vi "test - all.vi"() -> ()   [LabVIEW 2020]
uses:
  ui-testing.lvlib
panel:
  in  "Start test14 (SSP)":bool
  in  "Start test14 (SP)":bool
  in  "Start test14":bool
  in  "Start test13":bool
  in  "Start test12":bool
  in  "Start test11":bool
  in  "Start test10":bool
  in  "Start test9":bool
  in  "Start test8":bool
  in  "Start test7":bool
  in  "Start test6":bool
  in  "Start test5":bool
  in  "Start test4b":bool
  in  "Start test4":bool
  in  "Start test3":bool
  in  "Start test2":bool
  in  "Start test1":bool
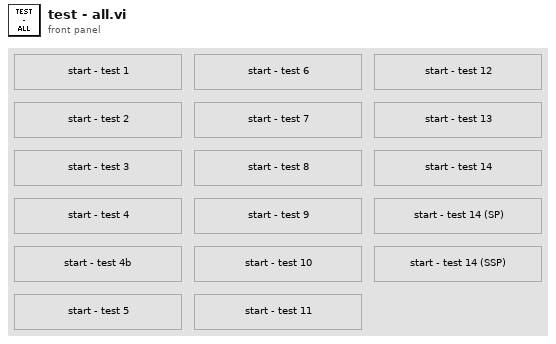
[diagram p1: front panel]
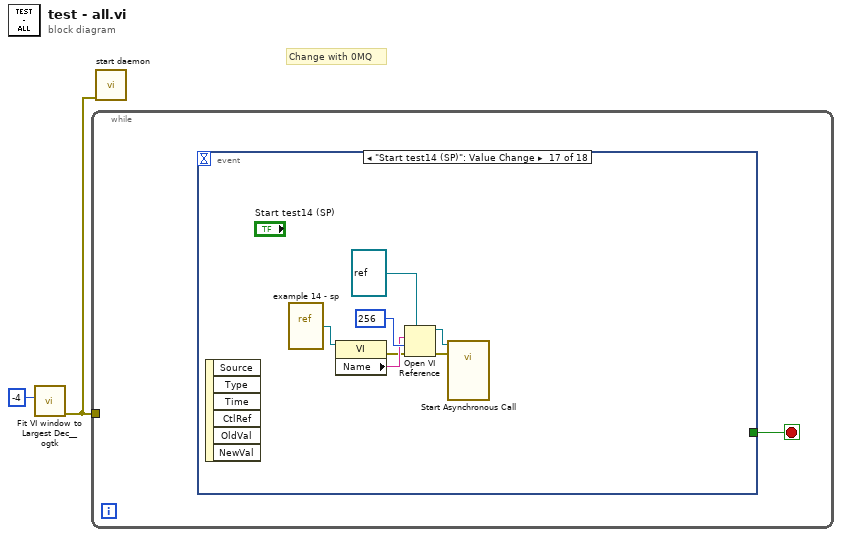
[diagram p0: block diagram]
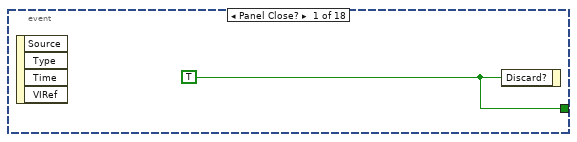
[diagram p2: hidden frame]
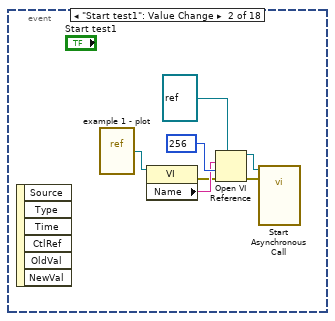
[diagram p3: hidden frame]
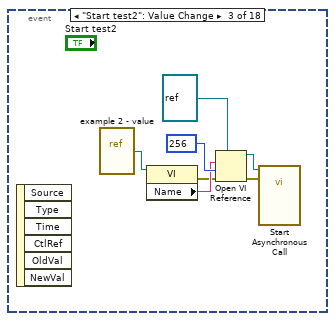
[diagram p4: hidden frame]
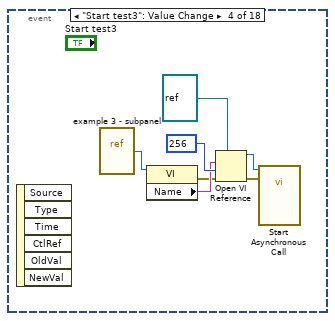
[diagram p5: hidden frame]
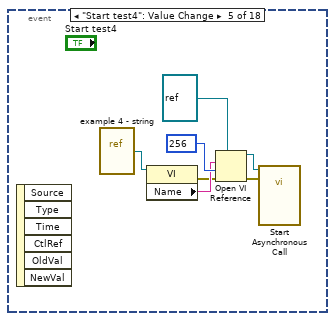
[diagram p6: hidden frame]
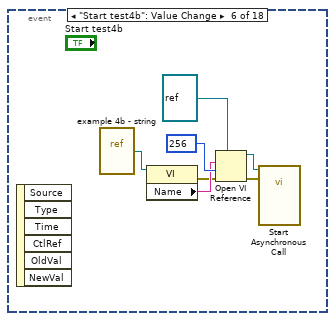
[diagram p7: hidden frame]
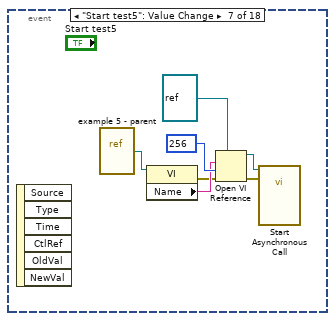
[diagram p8: hidden frame]
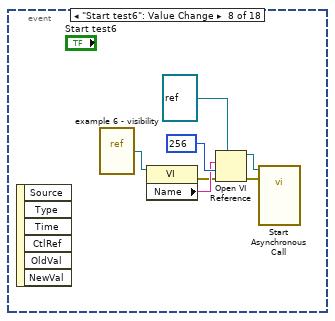
[diagram p9: hidden frame]
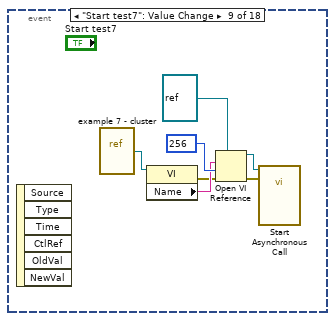
[diagram p10: hidden frame]
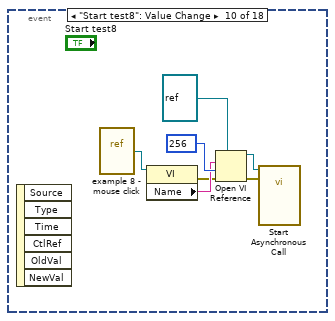
[diagram p11: hidden frame]
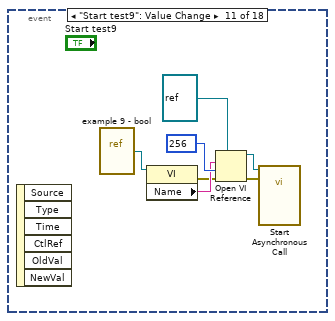
[diagram p12: hidden frame]
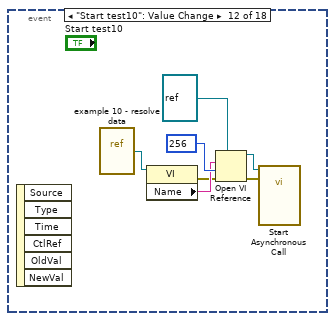
[diagram p13: hidden frame]
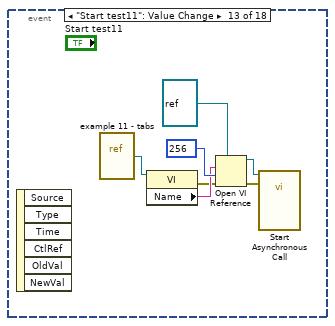
[diagram p14: hidden frame]
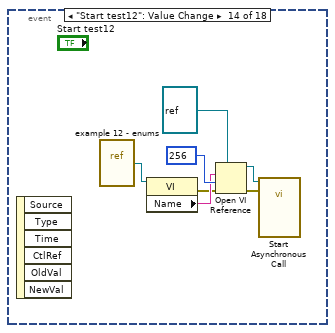
[diagram p15: hidden frame]
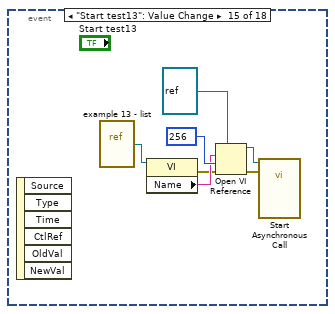
[diagram p16: hidden frame]
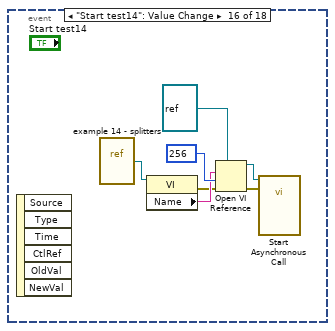
[diagram p17: hidden frame]
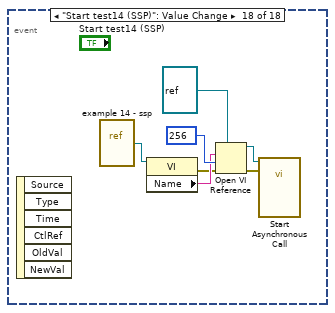
[diagram p18: hidden frame]
diagram:
  # "Change with 0MQ"
  n1 = call <userlib>:"Fit VI window to Largest Dec__ogtk.vi"("border spacing (2 px)"=-4) -> ("error out"=w1:errorcluster)  [unwired: 5 in, 1 out]
  n2 = while {
    tunnel: w1 -> [_]
    stop <- w3 stop-if-true
    n3 = event shown="[16] \"Start test14 (SP)\": Value Change" {
      selector: _ -> [_ _ _ _ _ _ _ _ _ _ _ _ _ _ _ _ _ _]
      dyn-events: _ -> [_ _ _ _ _ _ _ _ _ _ _ _ _ _ _ _ _ _]
      timeout: _ -> [_ _ _ _ _ _ _ _ _ _ _ _ _ _ _ _ _ _]
      tunnel: [w4 _ _ _ _ _ _ _ _ _ _ _ _ _ _ _ _ _] -> w3
      event Panel Close? {
        w4 = TRUE
        n4 = event-data() -> ()  [unwired: 1 in, 4 out]
        n5 = event-data("Discard?"=w4) -> ()  [unwired: 1 in, 1 out]
      }
      event "Start test1": Value Change {
        n6 = event-data() -> ()  [unwired: 1 in, 6 out]
        n7 = vi-ref "example 1 - plot.vi"() -> (w7:refnum<vi>)
        n8 = property class="VI"(reference=w7) -> (error out=w5:errorcluster, "Name"=w6:string)  [unwired: 1 in, 1 out]
        n9 = Open VI Reference(type specifier VI Refnum (for type only)=refnum<vi> refnum, vi path=w6, options=256 ("call and forget"), error in (no error)=w5) -> (vi reference=w9:refnum<vi>, error out=w8:errorcluster)  [unwired: 2 in]
        n10 = call-by-ref "Start Asynchronous Call"(reference=w9, error in=w8) -> ()  [unwired: 12 in, 2 out]
      }
      event "Start test2": Value Change {
        n11 = event-data() -> ()  [unwired: 1 in, 6 out]
        n12 = vi-ref "example 2 - value.vi"() -> (w14:refnum<vi>)
        n13 = property class="VI"(reference=w14) -> (error out=w12:errorcluster, "Name"=w13:string)  [unwired: 1 in, 1 out]
        n14 = Open VI Reference(type specifier VI Refnum (for type only)=refnum<vi> refnum, vi path=w13, options=256 ("call and forget"), error in (no error)=w12) -> (vi reference=w16:refnum<vi>, error out=w15:errorcluster)  [unwired: 2 in]
        n15 = call-by-ref "Start Asynchronous Call"(reference=w16, error in=w15) -> ()  [unwired: 12 in, 2 out]
      }
      event "Start test3": Value Change {
        n16 = event-data() -> ()  [unwired: 1 in, 6 out]
        n17 = vi-ref "example 3 - subpanel.vi"() -> (w21:refnum<vi>)
        n18 = property class="VI"(reference=w21) -> (error out=w19:errorcluster, "Name"=w20:string)  [unwired: 1 in, 1 out]
        n19 = Open VI Reference(type specifier VI Refnum (for type only)=refnum<vi> refnum, vi path=w20, options=256 ("call and forget"), error in (no error)=w19) -> (vi reference=w23:refnum<vi>, error out=w22:errorcluster)  [unwired: 2 in]
        n20 = call-by-ref "Start Asynchronous Call"(reference=w23, error in=w22) -> ()  [unwired: 12 in, 2 out]
      }
      event "Start test4": Value Change {
        n21 = event-data() -> ()  [unwired: 1 in, 6 out]
        n22 = vi-ref "example 4 - string.vi"() -> (w28:refnum<vi>)
        n23 = property class="VI"(reference=w28) -> (error out=w26:errorcluster, "Name"=w27:string)  [unwired: 1 in, 1 out]
        n24 = Open VI Reference(type specifier VI Refnum (for type only)=refnum<vi> refnum, vi path=w27, options=256 ("call and forget"), error in (no error)=w26) -> (vi reference=w30:refnum<vi>, error out=w29:errorcluster)  [unwired: 2 in]
        n25 = call-by-ref "Start Asynchronous Call"(reference=w30, error in=w29) -> ()  [unwired: 12 in, 2 out]
      }
      event "Start test4b": Value Change {
        n26 = event-data() -> ()  [unwired: 1 in, 6 out]
        n27 = vi-ref "example 4b - string.vi"() -> (w35:refnum<vi>)
        n28 = property class="VI"(reference=w35) -> (error out=w33:errorcluster, "Name"=w34:string)  [unwired: 1 in, 1 out]
        n29 = Open VI Reference(type specifier VI Refnum (for type only)=refnum<vi> refnum, vi path=w34, options=256 ("call and forget"), error in (no error)=w33) -> (vi reference=w37:refnum<vi>, error out=w36:errorcluster)  [unwired: 2 in]
        n30 = call-by-ref "Start Asynchronous Call"(reference=w37, error in=w36) -> ()  [unwired: 12 in, 2 out]
      }
      event "Start test5": Value Change {
        n31 = event-data() -> ()  [unwired: 1 in, 6 out]
        n32 = vi-ref "example 5 - parent.vi"() -> (w42:refnum<vi>)
        n33 = property class="VI"(reference=w42) -> (error out=w40:errorcluster, "Name"=w41:string)  [unwired: 1 in, 1 out]
        n34 = Open VI Reference(type specifier VI Refnum (for type only)=refnum<vi> refnum, vi path=w41, options=256 ("call and forget"), error in (no error)=w40) -> (vi reference=w44:refnum<vi>, error out=w43:errorcluster)  [unwired: 2 in]
        n35 = call-by-ref "Start Asynchronous Call"(reference=w44, error in=w43) -> ()  [unwired: 12 in, 2 out]
      }
      event "Start test6": Value Change {
        n36 = event-data() -> ()  [unwired: 1 in, 6 out]
        n37 = vi-ref "example 6 - visibility.vi"() -> (w49:refnum<vi>)
        n38 = property class="VI"(reference=w49) -> (error out=w47:errorcluster, "Name"=w48:string)  [unwired: 1 in, 1 out]
        n39 = Open VI Reference(type specifier VI Refnum (for type only)=refnum<vi> refnum, vi path=w48, options=256 ("call and forget"), error in (no error)=w47) -> (vi reference=w51:refnum<vi>, error out=w50:errorcluster)  [unwired: 2 in]
        n40 = call-by-ref "Start Asynchronous Call"(reference=w51, error in=w50) -> ()  [unwired: 12 in, 2 out]
      }
      event "Start test7": Value Change {
        n41 = event-data() -> ()  [unwired: 1 in, 6 out]
        n42 = vi-ref "example 7 - cluster.vi"() -> (w56:refnum<vi>)
        n43 = property class="VI"(reference=w56) -> (error out=w54:errorcluster, "Name"=w55:string)  [unwired: 1 in, 1 out]
        n44 = Open VI Reference(type specifier VI Refnum (for type only)=refnum<vi> refnum, vi path=w55, options=256 ("call and forget"), error in (no error)=w54) -> (vi reference=w58:refnum<vi>, error out=w57:errorcluster)  [unwired: 2 in]
        n45 = call-by-ref "Start Asynchronous Call"(reference=w58, error in=w57) -> ()  [unwired: 12 in, 2 out]
      }
      event "Start test8": Value Change {
        n46 = event-data() -> ()  [unwired: 1 in, 6 out]
        n47 = vi-ref "example 8 - mouse click.vi"() -> (w63:refnum<vi>)
        n48 = property class="VI"(reference=w63) -> (error out=w61:errorcluster, "Name"=w62:string)  [unwired: 1 in, 1 out]
        n49 = Open VI Reference(type specifier VI Refnum (for type only)=refnum<vi> refnum, vi path=w62, options=256 ("call and forget"), error in (no error)=w61) -> (vi reference=w65:refnum<vi>, error out=w64:errorcluster)  [unwired: 2 in]
        n50 = call-by-ref "Start Asynchronous Call"(reference=w65, error in=w64) -> ()  [unwired: 12 in, 2 out]
      }
      event "Start test9": Value Change {
        n51 = event-data() -> ()  [unwired: 1 in, 6 out]
        n52 = vi-ref "example 9 - bool.vi"() -> (w70:refnum<vi>)
        n53 = property class="VI"(reference=w70) -> (error out=w68:errorcluster, "Name"=w69:string)  [unwired: 1 in, 1 out]
        n54 = Open VI Reference(type specifier VI Refnum (for type only)=refnum<vi> refnum, vi path=w69, options=256 ("call and forget"), error in (no error)=w68) -> (vi reference=w72:refnum<vi>, error out=w71:errorcluster)  [unwired: 2 in]
        n55 = call-by-ref "Start Asynchronous Call"(reference=w72, error in=w71) -> ()  [unwired: 12 in, 2 out]
      }
      event "Start test10": Value Change {
        n56 = event-data() -> ()  [unwired: 1 in, 6 out]
        n57 = vi-ref "example 10 - resolve data.vi"() -> (w77:refnum<vi>)
        n58 = property class="VI"(reference=w77) -> (error out=w75:errorcluster, "Name"=w76:string)  [unwired: 1 in, 1 out]
        n59 = Open VI Reference(type specifier VI Refnum (for type only)=refnum<vi> refnum, vi path=w76, options=256 ("call and forget"), error in (no error)=w75) -> (vi reference=w79:refnum<vi>, error out=w78:errorcluster)  [unwired: 2 in]
        n60 = call-by-ref "Start Asynchronous Call"(reference=w79, error in=w78) -> ()  [unwired: 12 in, 2 out]
      }
      event "Start test11": Value Change {
        n61 = event-data() -> ()  [unwired: 1 in, 6 out]
        n62 = vi-ref "example 11 - tabs.vi"() -> (w84:refnum<vi>)
        n63 = property class="VI"(reference=w84) -> (error out=w82:errorcluster, "Name"=w83:string)  [unwired: 1 in, 1 out]
        n64 = Open VI Reference(type specifier VI Refnum (for type only)=refnum<vi> refnum, vi path=w83, options=256 ("call and forget"), error in (no error)=w82) -> (vi reference=w86:refnum<vi>, error out=w85:errorcluster)  [unwired: 2 in]
        n65 = call-by-ref "Start Asynchronous Call"(reference=w86, error in=w85) -> ()  [unwired: 12 in, 2 out]
      }
      event "Start test12": Value Change {
        n66 = event-data() -> ()  [unwired: 1 in, 6 out]
        n67 = vi-ref "example 12 - enums.vi"() -> (w91:refnum<vi>)
        n68 = property class="VI"(reference=w91) -> (error out=w89:errorcluster, "Name"=w90:string)  [unwired: 1 in, 1 out]
        n69 = Open VI Reference(type specifier VI Refnum (for type only)=refnum<vi> refnum, vi path=w90, options=256 ("call and forget"), error in (no error)=w89) -> (vi reference=w93:refnum<vi>, error out=w92:errorcluster)  [unwired: 2 in]
        n70 = call-by-ref "Start Asynchronous Call"(reference=w93, error in=w92) -> ()  [unwired: 12 in, 2 out]
      }
      event "Start test13": Value Change {
        n71 = event-data() -> ()  [unwired: 1 in, 6 out]
        n72 = vi-ref "example 13 - list.vi"() -> (w98:refnum<vi>)
        n73 = property class="VI"(reference=w98) -> (error out=w96:errorcluster, "Name"=w97:string)  [unwired: 1 in, 1 out]
        n74 = Open VI Reference(type specifier VI Refnum (for type only)=refnum<vi> refnum, vi path=w97, options=256 ("call and forget"), error in (no error)=w96) -> (vi reference=w100:refnum<vi>, error out=w99:errorcluster)  [unwired: 2 in]
        n75 = call-by-ref "Start Asynchronous Call"(reference=w100, error in=w99) -> ()  [unwired: 12 in, 2 out]
      }
      event "Start test14": Value Change {
        n76 = event-data() -> ()  [unwired: 1 in, 6 out]
        n77 = vi-ref "example 14 - splitters.vi"() -> (w105:refnum<vi>)
        n78 = property class="VI"(reference=w105) -> (error out=w103:errorcluster, "Name"=w104:string)  [unwired: 1 in, 1 out]
        n79 = Open VI Reference(type specifier VI Refnum (for type only)=refnum<vi> refnum, vi path=w104, options=256 ("call and forget"), error in (no error)=w103) -> (vi reference=w107:refnum<vi>, error out=w106:errorcluster)  [unwired: 2 in]
        n80 = call-by-ref "Start Asynchronous Call"(reference=w107, error in=w106) -> ()  [unwired: 12 in, 2 out]
      }
      event "Start test14 (SP)": Value Change {
        n81 = event-data() -> ()  [unwired: 1 in, 6 out]
        n82 = vi-ref "example 14 - sp.vi"() -> (w112:refnum<vi>)
        n83 = property class="VI"(reference=w112) -> (error out=w110:errorcluster, "Name"=w111:string)  [unwired: 1 in, 1 out]
        n84 = Open VI Reference(type specifier VI Refnum (for type only)=refnum<vi> refnum, vi path=w111, options=256 ("call and forget"), error in (no error)=w110) -> (vi reference=w114:refnum<vi>, error out=w113:errorcluster)  [unwired: 2 in]
        n85 = call-by-ref "Start Asynchronous Call"(reference=w114, error in=w113) -> ()  [unwired: 12 in, 2 out]
      }
      event "Start test14 (SSP)": Value Change {
        n86 = event-data() -> ()  [unwired: 1 in, 6 out]
        n87 = vi-ref "example 14 - ssp.vi"() -> (w119:refnum<vi>)
        n88 = property class="VI"(reference=w119) -> (error out=w117:errorcluster, "Name"=w118:string)  [unwired: 1 in, 1 out]
        n89 = Open VI Reference(type specifier VI Refnum (for type only)=refnum<vi> refnum, vi path=w118, options=256 ("call and forget"), error in (no error)=w117) -> (vi reference=w121:refnum<vi>, error out=w120:errorcluster)  [unwired: 2 in]
        n90 = call-by-ref "Start Asynchronous Call"(reference=w121, error in=w120) -> ()  [unwired: 12 in, 2 out]
      }
    }
  }
  n91 = call "start daemon.vi"("error in (no error)"=w1) -> ()  [unwired: 10 in, 1 out]
